vi "ampere.vi"(5 "divider":dbl, 6 "gain":enum16{"10x", "200x"}(ring), 7 "voltage \nreferences":enum16{"2,56", "5,00"}(ring), 8 "id pin":enum16{"ADC1/0 ", "ADC3/2"}(ring), 9 "connection in":refnum<k31>) -> (0 "reapons char error":errorcluster, 1 "ampere":dbl, 2 "check buffer error":errorcluster, 3 "connection out":refnum<k31>, 4 "sending error":errorcluster)   [LabVIEW 2012]
uses:
  meas_date.vi
panel:
  out "check buffer error 2":errorcluster
  out "income command id":u8
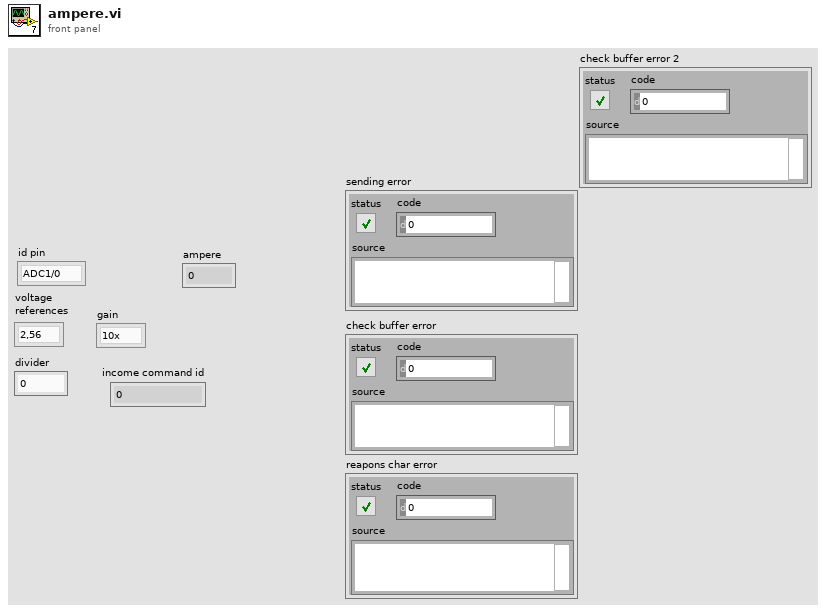
[diagram p1: front panel]
types:
  T1 = cluster{"param":u64, "count":i32, "name":string}[]
  T2 = cluster{"id":u8, "name":string, "params":cluster{"name":string, "count":u8}[], "respons char":string[]}[]
  T3 = cluster{"received values[0]":u8, "received values[1]":u8, "received values[2]":u8, "received values[3]":u8, "received values[4]":u8, "received values[5]":u8, "received values[6]":u8, "received values[7]":u8, "received values[8]":u8}
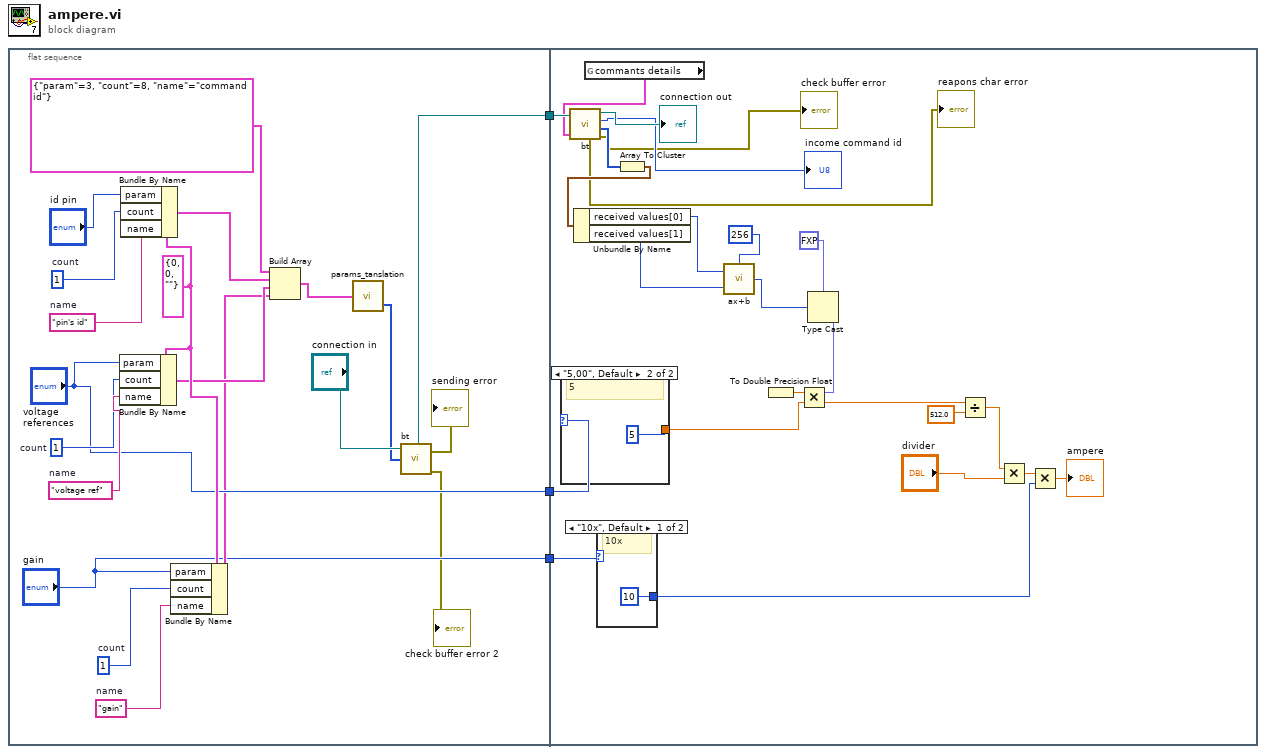
[diagram p0: block diagram]
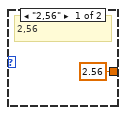
[diagram p2: hidden frame]
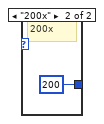
[diagram p3: hidden frame]
diagram:
  n1 = flat-sequence {
    tunnel: [w18] -> w3
    tunnel: ["gain"] -> w2
    tunnel: ["voltage \nreferences"] -> w1
    tunnel: w3 -> [w48]
    tunnel: w2 -> [w40]
    tunnel: w1 -> [w38]
    frame #0 {
      w14 = 1  # count
      w15 = "gain"  # name
      w16 = 1  # count
      w17 = "voltage ref"  # name
      w21 = 1  # count
      w22 = "pin's id"  # name
      w13 = cluster{"param":u64, "count":u8, "name":string} {"param"=0, "count"=0, "name"=""} ("Cluster")
      n2 = Bundle By Name(cluster=w13, "param"="voltage \nreferences", "count"=w16, "name"=w17) -> (w10:cluster{"param":u64, "count":u8, "name":string})
      n3 = Bundle By Name(cluster=w13, "param"="id pin", "count"=w21, "name"=w22) -> (w11:cluster{"param":u64, "count":u8, "name":string})
      n4 = Bundle By Name(cluster=w13, "param"="gain", "count"=w14, "name"=w15) -> (w9:cluster{"param":u64, "count":u8, "name":string})
      n5 = Build Array(cluster{"param":i32, "count":i32, "name":string} {"param"=3, "count"=8, "name"="command id"} ("Cluster"), w11, w10, w9) -> (w8:T1)
      n6 = call "params_tanslation.vi"("params"=w8) -> ("tablica charow (u8)"=w19:u8[])  [unwired: 1 out]
      n7 = call "bt.vi"("sending command"=w19, "connection in"="connection in") -> ("check buffer error"=→"check buffer error 2":errorcluster, "sending error"=→"sending error":errorcluster, "connection out"=w18:refnum<k31>)  [unwired: 1 in, 3 out]
    }
    frame #1 {
      n8 = case shown="\"5,00\", Default" w38 {
        tunnel: [2.56 5] -> w36
        frame "2,56" {
          # "2,56"
        }
        frame "5,00", Default {
          # "5"
        }
      }
      n9 = global read "meas_date.vi" "commants details"() -> (w24:T2)
      n10 = call "bt.vi"("commants details"=w24, "connection in"=w48) -> ("check buffer error"=→"check buffer error":errorcluster, "reapons char error"=→"reapons char error":errorcluster, "received values"=w44:u8[], "income command id"=→"income command id":u8, "connection out"=→"connection out":refnum<k31>)  [unwired: 1 in, 1 out]
      n11 = case shown="\"10x\", Default" w40 {
        tunnel: [10 200] -> w39
        frame "10x", Default {
          # "10x"
        }
        frame "200x" {
          # "200x"
        }
      }
      n12 = Array To Cluster(array=w44) -> (cluster=w45:T3)
      n13 = Unbundle By Name(w45) -> ("received values[0]"=w32:u8, "received values[1]"=w31:u8)
      n14 = call "ax+b.vi"("x"=256, "b"=w31, "a"=w32) -> ("y"=w26:i32)
      n15 = Type Cast(type=fxp<+/-,10,10> 0.0, x=w26) -> (*(type *) &x=w27:fxp<+/-,10,10>)
      n16 = To Double Precision Float(number=w27) -> (double precision float=w37:dbl)
      n17 = Multiply(x=w37, y=w36) -> (x*y=w35:dbl)
      n18 = Divide(x=w35, y=512.0) -> (x/y=w33:dbl)
      n19 = Multiply(x=w33, y="divider") -> (x*y=w42:dbl)
      n20 = Multiply(x=w42, y=w39) -> (x*y=→"ampere":dbl)
    }
  }
